vi "updateVariantDouble.vi"(8 "error in (no error)":errorcluster, 9 "variableName":string="BeamCentX", 10 "variantAttrribute":string="Beam_Center_X", 11 "variant":variant) -> (0 "error out":errorcluster, 3 "duplicate variant":variant)   [LabVIEW 2020, in "ThorlabsWavefrontDS.lvclass"]
uses:
  ThorlabsWavefrontDS.lvclass
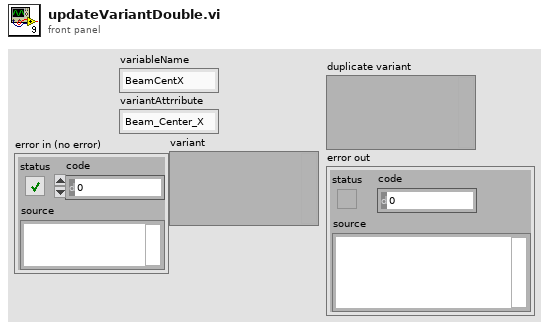
[diagram p1: front panel]
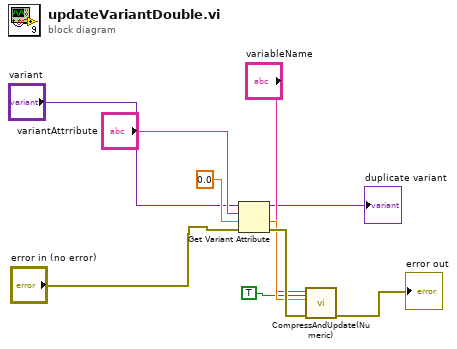
[diagram p0: block diagram]
diagram:
  n1 = Get Variant Attribute(Variant="variant", name="variantAttrribute", default value (empty Variant)=0.0, error in="error in (no error)") -> (duplicate Variant=→"duplicate variant":variant, value=w7:dbl, error out=w10:errorcluster)  [unwired: 1 out]
  n2 = call "CompressAndUpdate(Numeric).vi"("force CVT update (false)"=TRUE, "error in"=w10, "Numeric"=w7, "command or variable name"="variableName") -> ("error out"=→"error out":errorcluster)  [unwired: 7 in]
